vi "TRACE.vi"(7 "Mode":T1(ring), 9 "Parameter String":string, 10 "Function":string, 11 "TraceFile":path) -> ()   [LabVIEW 2009, in "POLARIS BME DG.lvlib"]
uses:
  POLARIS BME DG.lvlib
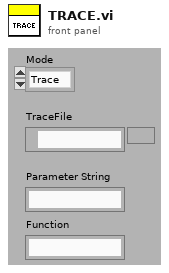
[diagram p1: front panel]
types:
  T1 = enum16{"Trace", "SetPath", "WriteToFile", "StopTrace"}
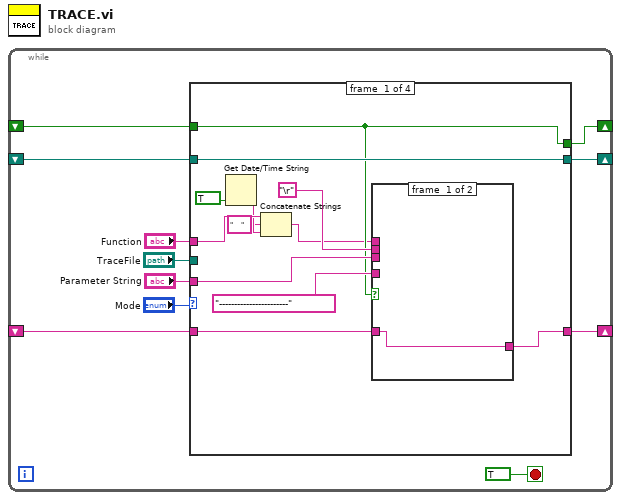
[diagram p0: block diagram]
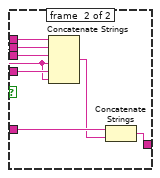
[diagram p2: hidden frame]
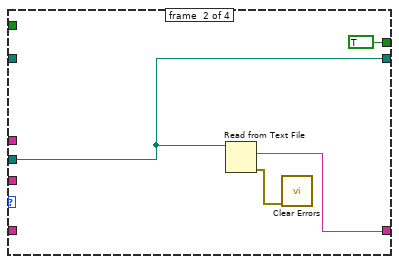
[diagram p3: hidden frame]
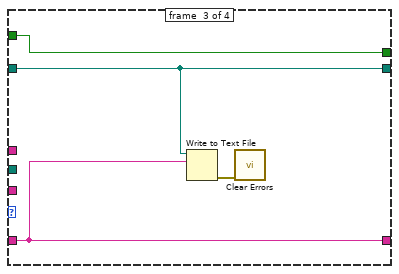
[diagram p4: hidden frame]
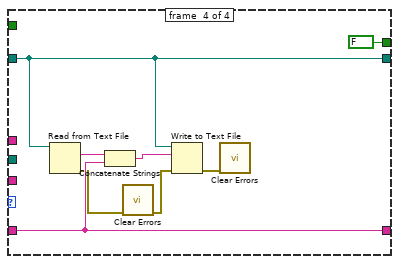
[diagram p5: hidden frame]
diagram:
  n1 = while {
    shift-right: [w9] -> _
    shift-left: _ -> [w7]
    shift-right: [w6] -> _
    shift-left: _ -> [w5]
    shift-right: [w4] -> _
    shift-left: _ -> [w3]
    stop <- TRUE stop-if-true
    n2 = case shown="\"Trace\", Default" "Mode" {
      tunnel: [w23 w34 w36 w45] -> w9
      tunnel: "TraceFile" -> [_ w34 _ _]
      tunnel: w7 -> [w23 _ w36 w45]
      tunnel: [w17 TRUE w39 FALSE] -> w6
      tunnel: w5 -> [w17 _ w39 _]
      tunnel: [w18 w32 w37 w46] -> w4
      tunnel: w3 -> [w19 _ w37 w46]
      tunnel: "Function" -> [w16 _ _ _]
      tunnel: "Parameter String" -> [w22 _ _ _]
      frame #0 {
        n3 = Get Date/Time String(want seconds? (F)=TRUE) -> (time string=w15:string)  [unwired: 2 in, 1 out]
        n4 = Concatenate Strings(w16, "    " ("string"), w15) -> (w12:string)
        n5 = case shown="True" w17 {
          tunnel: w12 -> [_ w31]
          tunnel: w22 -> [_ w30]
          tunnel: "-----------------------" ("string") -> [_ w29]
          tunnel: "\r" -> [_ w28]
          tunnel: w19 -> [w24 w27]
          tunnel: [w24 w25] -> w18
          frame #0 {
          }
          frame #1 {
            n6 = Concatenate Strings(w31, w28, w30, w28, w29, w28) -> (w26:string)
            n7 = Concatenate Strings(w27, w26) -> (w25:string)
          }
        }
      }
      frame #1 {
        n8 = Read from Text File(file (use dialog)=w34) -> (text=w32:string, error out=w33:errorcluster)  [unwired: 3 in, 2 out]
        n9 = call <vilib>:"Clear Errors.vi"("error in (no error)"=w33) -> ()  [unwired: 6 in, 1 out]
      }
      frame #2 {
        n10 = Write to Text File(file (use dialog)=w36, text=w37) -> (error out=w38:errorcluster)  [unwired: 2 in, 2 out]
        n11 = call <vilib>:"Clear Errors.vi"("error in (no error)"=w38) -> ()  [unwired: 6 in, 1 out]
      }
      frame #3 {
        n12 = Read from Text File(file (use dialog)=w45) -> (text=w44:string, error out=w41:errorcluster)  [unwired: 3 in, 2 out]
        n13 = Concatenate Strings(w44, w46) -> (w43:string)
        n14 = call <vilib>:"Clear Errors.vi"("error in (no error)"=w41) -> ("error out"=w40:errorcluster)  [unwired: 6 in]
        n15 = Write to Text File(file (use dialog)=w45, text=w43, error in=w40) -> (error out=w42:errorcluster)  [unwired: 1 in, 2 out]
        n16 = call <vilib>:"Clear Errors.vi"("error in (no error)"=w42) -> ()  [unwired: 6 in, 1 out]
      }
    }
  }
